vi "DN4_CheckSamplesCount.vi"(1 "samples count":i32) -> (0 "error out":errorcluster)   [LabVIEW 2020]
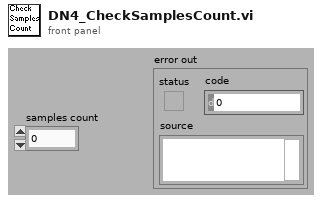
[diagram p1: front panel]
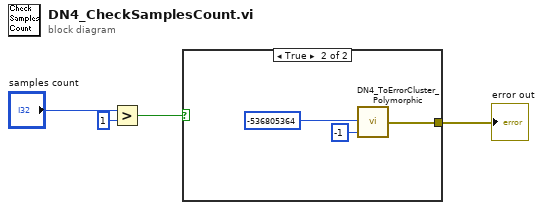
[diagram p0: block diagram]
diagram:
  n1 = Greater?(x="samples count", y=1) -> (0:w3:bool)
  n2 = case shown="True" w3 {
    tunnel: [_ w6] -> w4
    frame False {
    }
    frame True {
      n3 = call "DN4_ToErrorCluster_Polymorphic.vi"("task id"=-1, "error code"=-536805364 ("error code (0)")) -> ("error out"=w6:errorcluster)  [unwired: 3 out]
    }
  }
  "error out" <- w4
